vi "Find Workspace.vi"(6 "Pickup_Test_Number":dbl, 7 "Database Entry in":refnum<class "Database Entry.lvclass">, 8 "Error In":errorcluster, 9 "Assembly Type":string, 10 "Control In":T2={"I-O.lvclass"=refnum, "Gantry"=refnum, "Dispenser"="COM1"}, 11 "Workspace In":refnum<class "Current Position.lvclass">) -> (0 "Error Out":errorcluster, 1 "Workspace Out":T1, 2 "Control Out":T2={"I-O.lvclass"=refnum, "Gantry"=refnum, "Dispenser"="COM1"}, 3 "Workspace Out":refnum<class "Current Position.lvclass">, 5 "Database Entry out":refnum<class "Database Entry.lvclass">)   [LabVIEW 2021, in "Current Position.lvclass"]
uses:
  Current Position.lvclass
  Controller/Controllers.ctl
  Controller/I-O/I-O.lvclass
  C:/Program Files (x86)/Aerotech/A3200/LabVIEW/2010/Bin/Aerotech.A3200.dll
  Program Files (x86)/Aerotech/A3200/LabVIEW/2010/Bin/Aerotech.A3200.dll
  Workspace.ctl
  Assembly/Database Entry/Database Entry.lvclass
  Controller/Motion/Motion.lvclass
  Controller/Controller.lvclass
  Fixture.lvclass
panel:
  in  "Workspace":T1
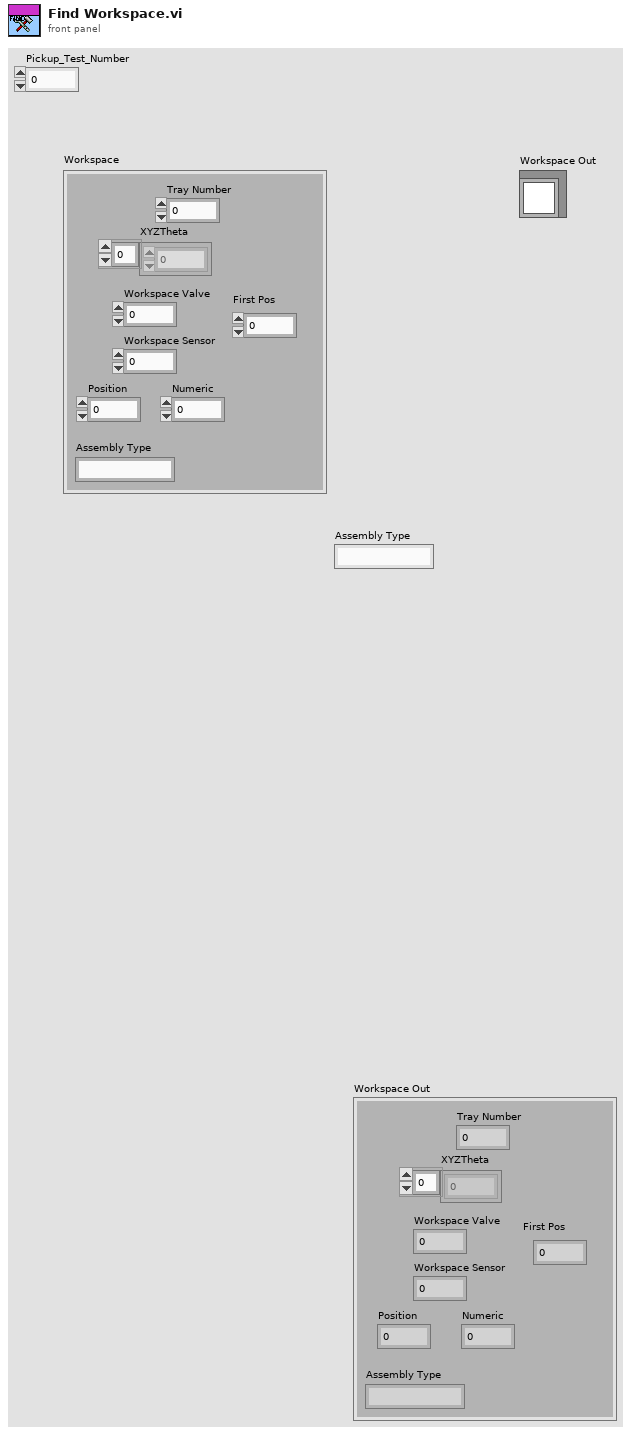
[diagram p1: front panel]
types:
  T1 = typedef "Fixture.lvclass/Workspace.ctl" = cluster{"XYZTheta":dbl[], "Workspace Valve":i32, "Workspace Sensor":i32, "Tray Number":i32, "Position":i32, "Assembly Type":string, "Numeric":dbl, "First Pos":i32}
  T2 = typedef "Controller.lvclass/Controllers.ctl" = cluster{"I-O.lvclass":refnum<class "I-O.lvclass">, "Gantry":refnum<k24>, "Dispenser":refnum<visa-resource-name>}
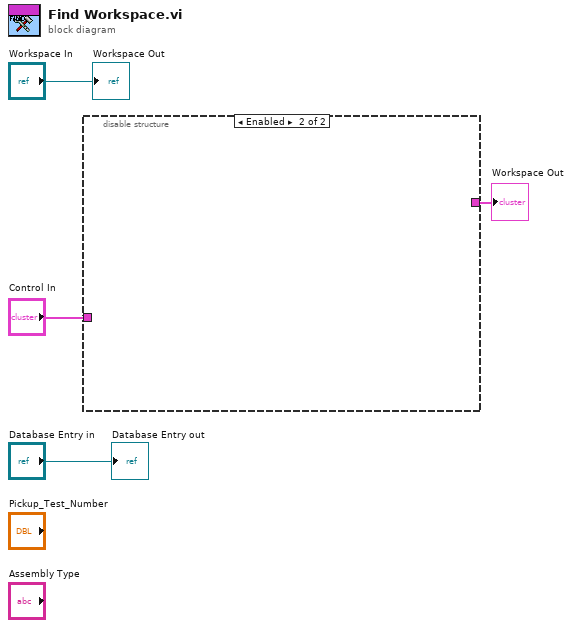
[diagram p0: block diagram]
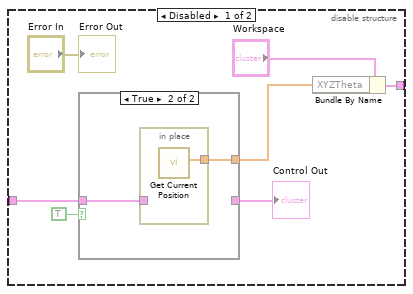
[diagram p2: hidden frame]
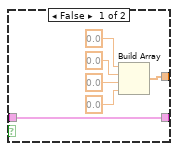
[diagram p3: hidden frame]
diagram:
  n1 = disable-structure shown="Enabled" {
    disable-tunnel: "Control In" -> [w11 _]
    disable-tunnel: [w7 _] -> w3
    frame Disabled {
      n2 = case shown="True" TRUE {
        tunnel: w11 -> [w17 w18]
        tunnel: [w17 _] -> w10
        tunnel: [w16 w19] -> w8
        frame False {
          n3 = Build Array(0.0, 0.0, 0.0, 0.0) -> (w16:dbl[])
        }
        frame True {
          n4 = in-place {
            in-place-border: [w20] -> w19
            in-place-border: w18 -> [_]
            n5 = call-dynamic "Get Current Position.vi"() -> ("XYZTheta Out"=w20:dbl[])  [unwired: 9 in, 2 out]
          }
        }
      }
      "Control Out" <- w10
      n6 = Bundle By Name(cluster="Workspace", "XYZTheta"=w8) -> (w7:T1)
      "Error Out" <- "Error In"
    }
    frame Enabled {
    }
  }
  "Workspace Out" <- w3
  "Workspace Out" <- "Workspace In"
  "Database Entry out" <- "Database Entry in"
